vi "Write AI to DMA FIFO.vi"(1 "Channel Scale Array":fxp<+,24,12>[](array[numeric])=[0.0, 0.0, 0.0, 0.0], 2 "Channel AI Array":fxp<+/-,24,4>[](array[numeric])=[0.0, 0.0, 0.0, 0.0]) -> (0 "Overflow Status":bool)   [LabVIEW 2013]
uses:
  <vilib>/rvi/interface/RandomDataEmulation/nirviRandomDataFPGAFIFO.vi
  <vilib>/rvi/interface/RandomDataEmulation/niFpgaRandomDataHandleErrors.vi
  <vilib>/rvi/DataTransferAndStorage/Container/XNode/niFpgaContainer.xnode
  <vilib>/rvi/interface/RandomDataEmulation/nirviRandomDataFpgaReadWriteTemplate.vi
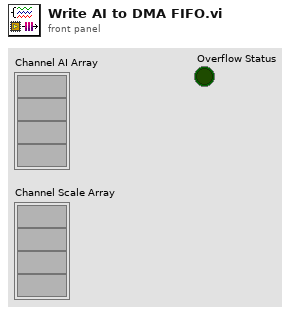
[diagram p1: front panel]
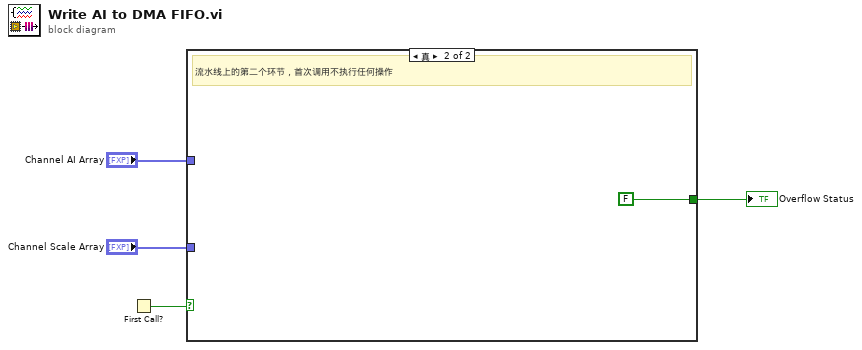
[diagram p0: block diagram]
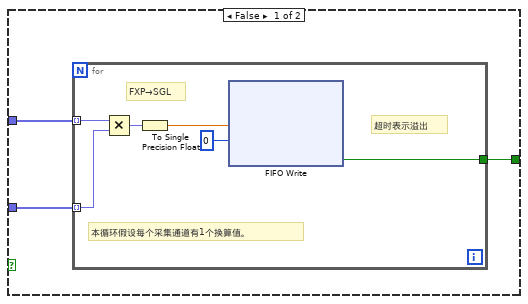
[diagram p2: hidden frame]
diagram:
  n1 = First Call?() -> (First Call?: T/F=w4:bool)
  n2 = case shown="真" w4 {
    tunnel: "Channel Scale Array" -> [w7 _]
    tunnel: "Channel AI Array" -> [w6 _]
    tunnel: [w5 FALSE] -> w1
    frame False {
      n3 = for {
        tunnel: [w13] -> w5
        tunnel: w6 -> [w11] mode=indexing
        tunnel: w7 -> [w10] mode=indexing
        # "本循环假设每个采集通道有1个换算值。"
        # "超时表示溢出"
        # "FXP→SGL"
        n4 = Multiply(x=w11, y=w10) -> (x*y=w9:fxp<+/-,48,16>)
        n5 = To Single Precision Float(number=w9) -> (single precision float=w8:sgl)
        n6 = xnode ("FIFO Write")("元素"=w8, "超时"=0) -> ("超时？"=w13:bool)  [unwired: 1 in, 1 out]
      }
    }
    frame True {
      # "流水线上的第二个环节，首次调用不执行任何操作"
    }
  }
  "Overflow Status" <- w1
